vi "Select Reference Human VOG.vi"(1 "3D Coil":dbl[][](graph)) -> (0 "References":i32[](array[numeric]))   [LabVIEW 2013]
panel:
  in  "HEAD":bool
  in  "LE":bool
  in  "RE":bool
  # "Copyright Americo A. Migliaccio (c) 2002 All Rights Reserved by Author"
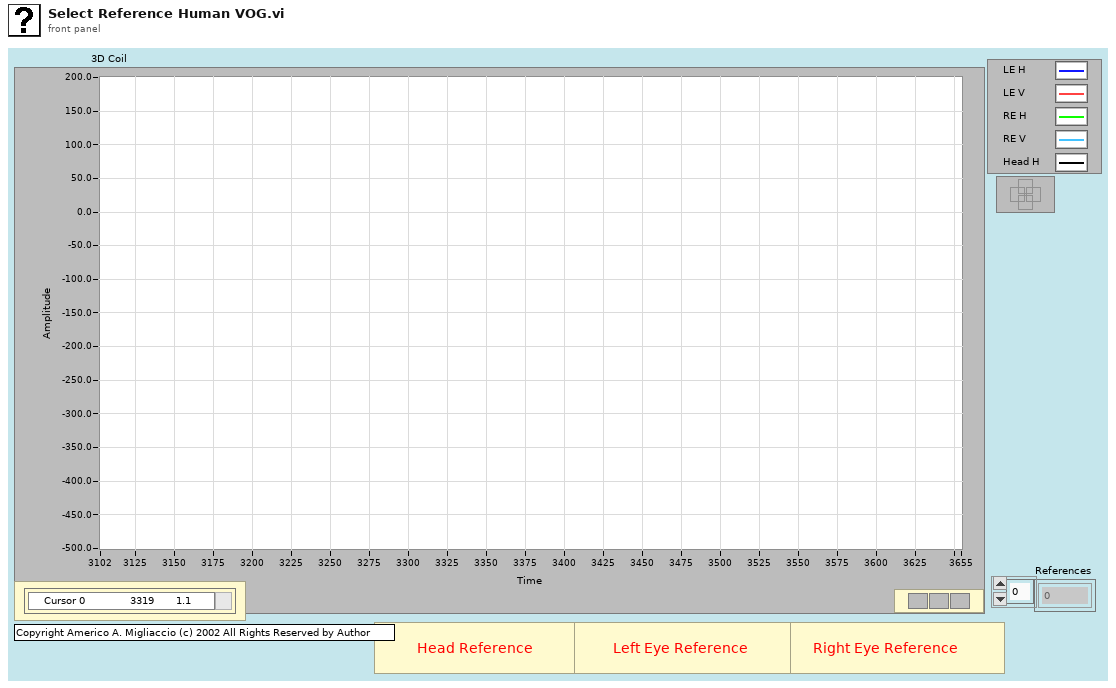
[diagram p1: front panel]
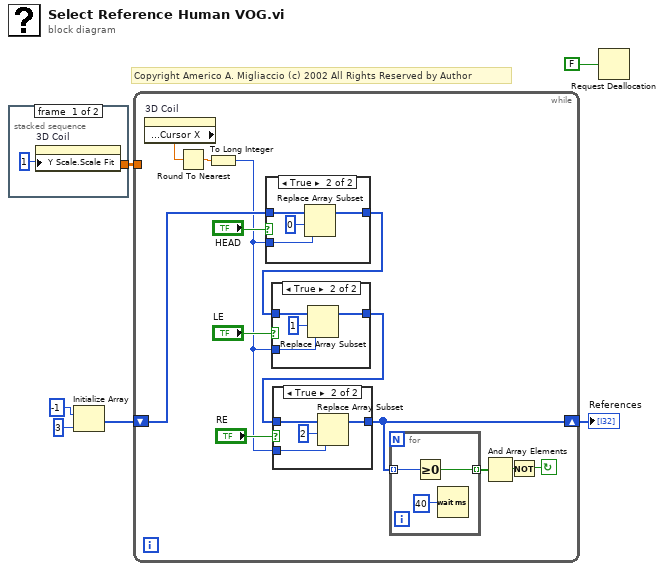
[diagram p0: block diagram]
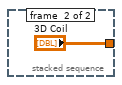
[diagram p5: hidden frame]
diagram:
  # "Copyright Americo A. Migliaccio (c) 2002 All Rights Reserved by Author"
  n1 = stacked-sequence {
    tunnel: [_ "3D Coil"] -> w6
    frame #0 {
      n2 = property on="3D Coil" class="WFGraph (strict)"("Y Scale.Scale Fit"=u8 1) -> ()  [unwired: 2 in, 2 out]
    }
    frame #1 {
    }
  }
  n3 = Initialize Array(-1 ("Element Data"), 3 ("Dimension Size")) -> (w5:i32[])
  n4 = while {
    shift-left: w5 -> [w17]
    shift-right: [w12] -> w2
    tunnel: w6 -> [_]
    stop <- w9 continue-if-true
    n5 = property on="3D Coil" class="WFGraph (strict)"() -> ("Cursor.Cursor Position:Cursor X"=w21:dbl)  [unwired: 2 in, 2 out]
    n6 = Round To Nearest(number=w21) -> (nearest integer value=w14:dbl)
    n7 = To Long Integer(number=w14) -> (32bit integer=w13:i32)
    n8 = case shown="True" "HEAD" {
      tunnel: w17 -> [w35 w38]
      tunnel: [w35 w37] -> w16
      tunnel: w13 -> [_ w36]
      frame False {
      }
      frame True {
        n9 = Replace Array Subset(array=w38, new element=w36, index=0 ("Index")) -> (w37:i32[])
      }
    }
    n10 = case shown="True" "LE" {
      tunnel: w16 -> [w30 w33]
      tunnel: [w30 w32] -> w15
      tunnel: w13 -> [_ w31]
      frame False {
      }
      frame True {
        n11 = Replace Array Subset(array=w33, new element=w31, index=1 ("Index")) -> (w32:i32[])
      }
    }
    n12 = case shown="True" "RE" {
      tunnel: w15 -> [w25 w28]
      tunnel: [w25 w27] -> w12
      tunnel: w13 -> [_ w26]
      frame False {
      }
      frame True {
        n13 = Replace Array Subset(array=w28, new element=w26, index=2 ("Index")) -> (w27:i32[])
      }
    }
    n14 = for {
      tunnel: w12 -> [w24] mode=indexing
      tunnel: [w23] -> w11 mode=indexing
      n15 = Greater Or Equal To 0?(x=w24) -> (x >= 0?=w23:bool)
      n16 = Wait (ms)(milliseconds to wait=u32 40) -> ()  [unwired: 1 out]
    }
    n17 = And Array Elements(Boolean array=w11) -> (logical AND=w10:bool)
    n18 = Not(x=w10) -> (.not. x?=w9:bool)
  }
  "References" <- w2
  n19 = Request Deallocation(FALSE ("flag")) -> ()
